vi "control_label_font.vi"(8 "error in (no error)":errorcluster, 11 "VI Ref In":refnum<vi>) -> (0 "error out":errorcluster, 3 "VI Ref Out":refnum<vi>)   [LabVIEW 2018]
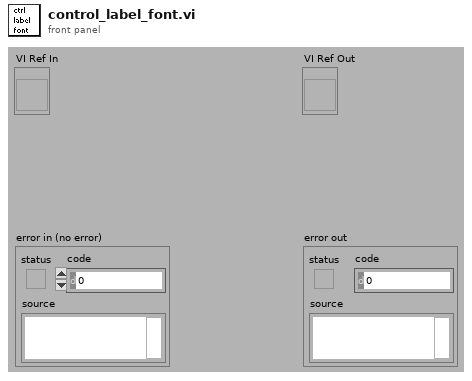
[diagram p1: front panel]
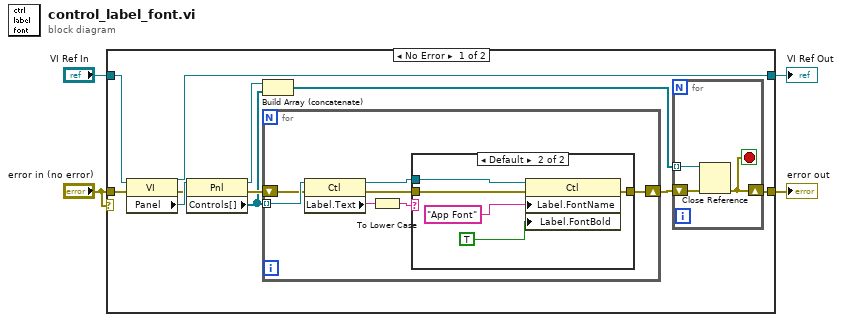
[diagram p0: block diagram]
diagram:
  n1 = case shown="No Error" "error in (no error)" {
    tunnel: [w8 w33] -> w4
    tunnel: "VI Ref In" -> [w7 w33]
    tunnel: "error in (no error)" -> [w6 w32]
    tunnel: [w5 w32] -> w2
    frame No Error {
      n2 = property class="VI"(reference=w7, error in=w6) -> (reference out=w8:refnum<vi>, error out=w14:errorcluster, "Panel"=w15:refnum<vi>)
      n3 = property class="Pnl"(reference=w15, error in=w14) -> (reference out=w12:refnum<vi>, error out=w13:errorcluster, "Controls[]"=w11:refnum<vi>[])
      n4 = Build Array (concatenate)(w12, w11) -> (w10:refnum<vi>[])
      n5 = for {
        tunnel: w11 -> [w23] mode=indexing
        shift-right: [w25] -> w9
        shift-left: w13 -> [w22]
        n6 = property class="Ctl"(reference=w23, error in=w22) -> (reference out=w21:refnum<vi>, error out=w24:errorcluster, "Label.Text"=w20:string)
        n7 = To Lower Case(string=w20) -> (all lower case string=w19:string)
        n8 = case shown="Default" w19 {
          tunnel: w24 -> [w26 w29]
          tunnel: [w26 w31] -> w25
          tunnel: w21 -> [_ w30]
          frame "error in (no error)" {
          }
          frame Default {
            n9 = property class="Ctl"(reference=w30, error in=w29, "Label.FontName"="App Font" ("Label.Font:Name"), "Label.FontBold"=TRUE ("Label.Font:Bold")) -> (error out=w31:errorcluster)  [unwired: 1 out]
          }
        }
      }
      n10 = for {
        tunnel: w10 -> [w18] mode=indexing
        shift-right: [w16] -> w5
        shift-left: w9 -> [w17]
        stop <- w16 stop-if-true
        n11 = Close Reference(reference=w18, error in (no error)=w17) -> (error out=w16:errorcluster)
      }
    }
    frame Error {
    }
  }
  "VI Ref Out" <- w4
  "error out" <- w2
